vi "XY Graph Update Plot & Style.vi"(4 "Y Array":dbl[](array[numeric]), 6 "X Array":dbl[](array[numeric]), 8 "Error In":errorcluster, 9 "XY Plot Properties":T1, 10 "Plot Idx":i32, 11 "XY Graph refnum":refnum<vi>) -> (0 "Error Out":errorcluster)   [LabVIEW 2019]
uses:
  XY Graph Plot Properties.ctl
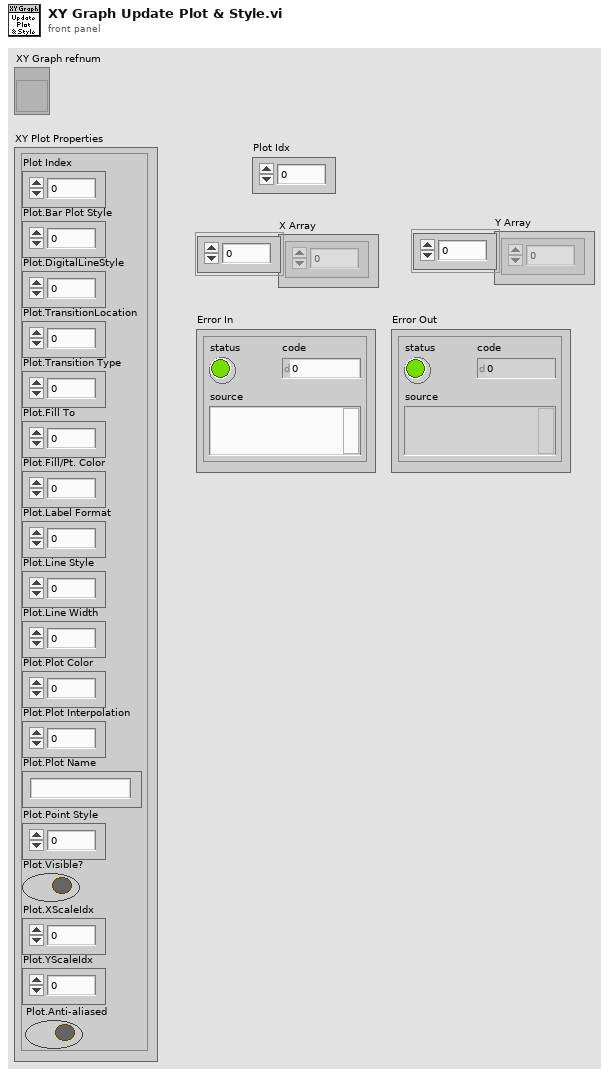
[diagram p1: front panel]
types:
  T1 = typedef "XY Graph Plot Properties.ctl" = cluster{"Plot Index":i32, "Plot.Bar Plot Style":u8, "Plot.DigitalLineStyle":u8, "Plot.TransitionLocation":u8, "Plot.Transition Type":u8, "Plot.Fill To":i16, "Plot.Fill/Pt. Color":u32, "Plot.Label Format":u8, "Plot.Line Style":u8, "Plot.Line Width":u8, "Plot.Plot Color":u32, "Plot.Plot Interpolation":u8, "Plot.Plot Name":string, "Plot.Point Style":u8, "Plot.Visible?":bool, "Plot.XScaleIdx":u32, "Plot.YScaleIdx":u32, "Plot.Anti-aliased":bool}
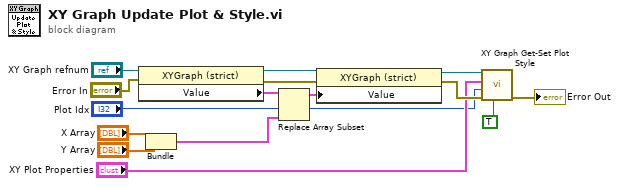
[diagram p0: block diagram]
diagram:
  n1 = property class="XYGraph (strict)"(reference="XY Graph refnum", error in="Error In") -> (reference out=w10:refnum<vi>, error out=w9:errorcluster, "Value"=w14:cluster{"X Array":dbl[], "Y Array":dbl[]}[])
  n2 = Bundle("X Array"="X Array", "Y Array"="Y Array") -> (w11:cluster{"X Array":dbl[], "Y Array":dbl[]})  [unwired: 1 in]
  n3 = Replace Array Subset(array=w14, new element=w11, index="Plot Idx") -> (w8:cluster{"X Array":dbl[], "Y Array":dbl[]}[])
  n4 = property class="XYGraph (strict)"(reference=w10, error in=w9, "Value"=w8) -> (reference out=w7:refnum<vi>, error out=w6:errorcluster)
  n5 = call "XY Graph Get-Set Plot Style.vi"("Get (F)/Set"=TRUE, "Error In"=w6, "Plot Index"="Plot Idx", "Plot Style in"="XY Plot Properties", "XYGraph in"=w7) -> ("Error Out"=→"Error Out":errorcluster)  [unwired: 3 in, 3 out]
